vi "Drag and Drop.vi"(8 "error in":errorcluster) -> (0 "error out":errorcluster)   [LabVIEW 2024]
doc: "This VI illustrates the use of a built-in Drag and Drop source with custom Drag and Drop data and a custom target. The specific events illustrated by this example are:\n\nDrag Starting? - Triggered when a drag begins. This is a source-side event. Drag Data is passed as an array of 2-element clusters containing a \"data name\" and variant \"drag data.\"\n\nDrag Enter - Triggered when a Drag and Drop enters any control or indicator. This is a target-side event. The Available Data Names are searched for a name that matches the expected data name. If a match is found the Drag enter is accepted and the cursor is changed to indicate that a valid drop target has been found.\n\nDrop - Triggered when a Drag and Drop ends within a control or indicator. This is a target-side event. A Drag and Drop \"data name\" and \"data type\" prototype are given to extract the original data from the array and convert from variant to the intended data type. The Get Drag Drop Data function is used for this process."
panel:
  in  "Clear":bool=TRUE
  in  "stop":bool
  out "Protocol":i32(listbox)=-1
  in  "Sequences":i32(listbox)=2
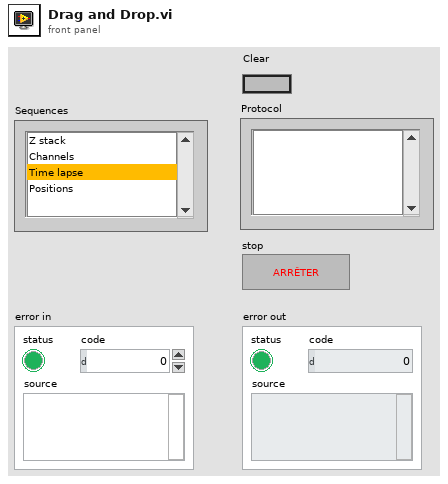
[diagram p1: front panel]
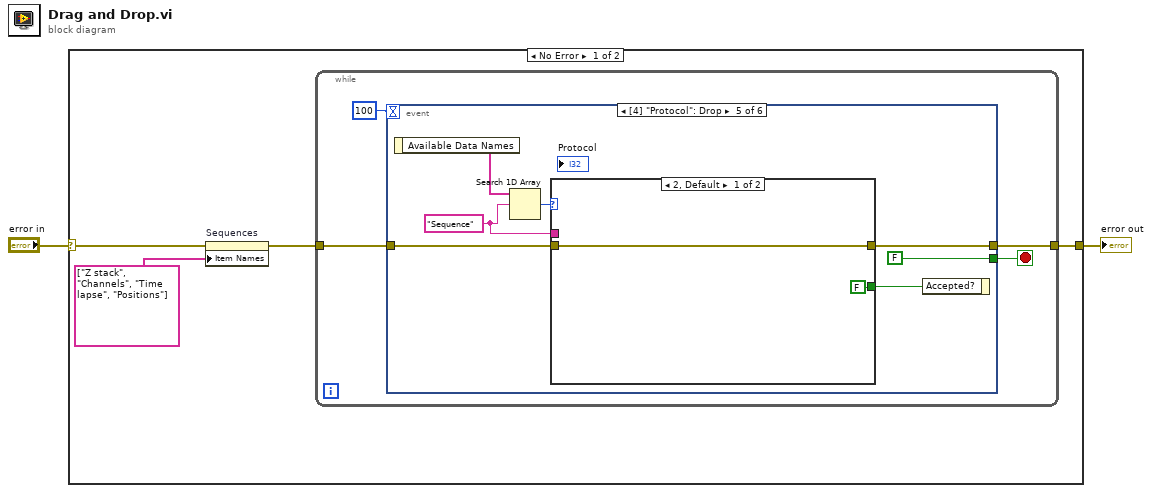
[diagram p0: block diagram]
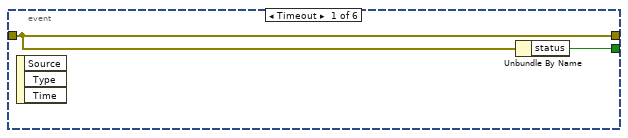
[diagram p2: hidden frame]
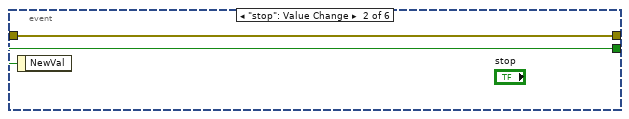
[diagram p3: hidden frame]
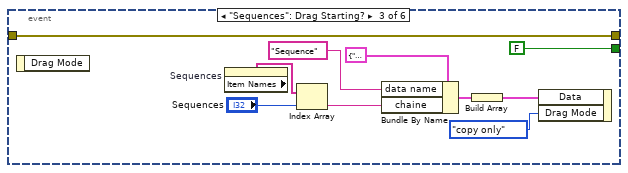
[diagram p4: hidden frame]
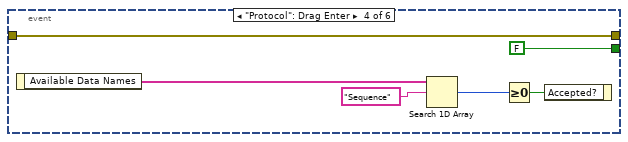
[diagram p5: hidden frame]
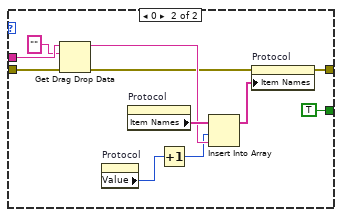
[diagram p6: hidden frame]
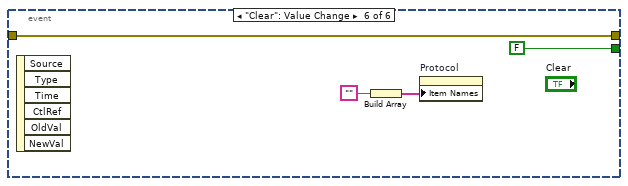
[diagram p7: hidden frame]
diagram:
  n1 = case shown="No Error" "error in" {
    selector: "error in" -> [w4 w55]
    tunnel: [w6 w55] -> w1
    frame No Error {
      n2 = property on="Sequences" class="LstBox (strict)"(error in=w4, "Item Names"=string[] ["Z stack", "Channels", "Time lapse", "Positions"]) -> (error out=w3:errorcluster)  [unwired: 1 in, 1 out]
      n3 = while {
        tunnel: [w8] -> w6
        tunnel: w3 -> [w7]
        stop <- w10 stop-if-true
        n4 = event shown="[4] \"Protocol\": Drop" {
          selector: _ -> [_ _ _ _ _ _]
          dyn-events: _ -> [_ _ _ _ _ _]
          timeout: 100 -> [_ _ _ _ _ _]
          tunnel: [w12 w14 FALSE ("stop") FALSE ("stop") FALSE ("stop") FALSE ("stop")] -> w10
          tunnel: [w11 w13 w16 w25 w32 w51] -> w8
          tunnel: w7 -> [w11 w13 w16 w25 w31 w51]
          event Timeout {
            n5 = event-data() -> ()  [unwired: 1 in, 3 out]
            n6 = Unbundle By Name(w11) -> ("status"=w12:bool)
          }
          event "stop": Value Change {
            n7 = event-data() -> ("NewVal"=w14:bool)  [unwired: 1 in]
          }
          event "Sequences": Drag Starting? {
            n8 = event-data ("Nœud de données d'événement")() -> ()  [unwired: 1 in, 1 out]
            n9 = property on="Sequences" class="LstBox (strict)"() -> ("Item Names"=w15:string[])  [unwired: 2 in, 2 out]
            n10 = Index Array(array=w15, index="Sequences") -> (element=w17:string)
            n11 = Bundle By Name(cluster=cluster{"data name":string, "chaine":string} {"data name"="", "chaine"=""} ("Cluster"), "data name"="Sequence", "chaine"=w17) -> (w21:cluster{"data name":string, "chaine":string})
            n12 = Build Array(w21) -> (w20:cluster{"data name":string, "chaine":string}[])
            n13 = event-data("Data"=w20, "Drag Mode"=enum32{"copy or move", "copy only", "move only"}."copy only" ("Mode de glissement")) -> ()  [unwired: 1 in, 1 out]
          }
          event "Protocol": Drag Enter {
            n14 = event-data ("Nœud de données d'événement")() -> ("Available Data Names"=w30:string[])  [unwired: 1 in]
            n15 = Search 1D Array(1D array=w30, element="Sequence" ("élément")) -> (index of element=w29:i32)  [unwired: 1 in]
            n16 = Greater Or Equal To 0?(x=w29) -> (x >= 0?=w28:bool)
            n17 = event-data("Accepted?"=w28) -> ()  [unwired: 1 in, 1 out]
          }
          event "Protocol": Drop {
            w35 = "Sequence" ("élément")
            n18 = event-data ("Nœud de données d'événement")() -> ("Available Data Names"=w37:string[])  [unwired: 1 in]
            n19 = Search 1D Array(1D array=w37, element=w35) -> (index of element=w36:i32)  [unwired: 1 in]
            n20 = case shown="2, Default" w36 {
              tunnel: w35 -> [_ w50]
              tunnel: [FALSE TRUE] -> w34
              tunnel: w31 -> [w38 w42]
              tunnel: [w38 w40] -> w32
              frame 2, Default {
              }
              frame 0 {
                n21 = Get Drag Drop Data(6:w42, 8:"" ("élément"), 9:w50) -> (0:w41:errorcluster, 3:w46:string)
                n22 = property on="Protocol" class="LstBox (strict)"() -> ("Value"=w45:i32)  [unwired: 2 in, 2 out]
                n23 = property on="Protocol" class="LstBox (strict)"() -> ("Item Names"=w47:string[])  [unwired: 2 in, 2 out]
                n24 = Increment(x=w45) -> (x+1=w44:i32)
                n25 = Insert Into Array(array=w47, index=w44, new element=w46) -> (w43:string[])
                n26 = property on="Protocol" class="LstBox (strict)"(error in=w41, "Item Names"=w43) -> (error out=w40:errorcluster)  [unwired: 1 in, 1 out]
              }
            }
            n27 = event-data("Accepted?"=w34) -> ()  [unwired: 1 in, 1 out]
          }
          event "Clear": Value Change {
            n28 = event-data ("Nœud de données d'événement")() -> ()  [unwired: 1 in, 6 out]
            n29 = Build Array("") -> (w53:string[])
            n30 = property on="Protocol" class="LstBox (strict)"("Item Names"=w53) -> ()  [unwired: 2 in, 2 out]
          }
        }
      }
    }
    frame Error {
    }
  }
  "error out" <- w1
